vi "Read Tab Size.vi"(9 "Tab in":refnum<class "Tab.lvclass">) -> (3 "Tab out":refnum<class "Tab.lvclass">, 4 "Tab Size":T1(ring))   [LabVIEW 2014, in "Tab.lvclass"]
uses:
  Tab.lvclass
  Tab.lvclass/Tab.ctl
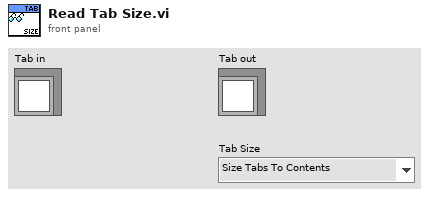
[diagram p1: front panel]
types:
  T1 = enum32{"Size Tabs To Contents", "Size All Tabs to Largest Tab", "Fixed Tab Size"}
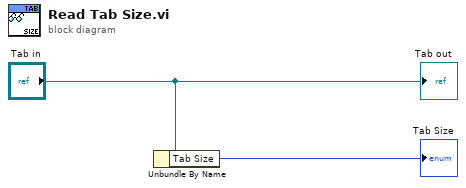
[diagram p0: block diagram]
diagram:
  n1 = Unbundle By Name("Tab in") -> ("Tab Size"=→"Tab Size":T1)
  "Tab out" <- "Tab in"
